vi "根据拍PCB孔点计算所有放料点.vi"(8 "放料点相对拍照点高度差(数组)":dbl[](array[numeric]), 9 "自动锁螺丝: 点位补偿值-单片PCB":T1[](array[typedef]), 11 "自动锁螺丝: PCB孔拍照点坐标-单片PCB":T2[](array[typedef])) -> (1 "放料点XYZ 数组":T1[](array[typedef]), 3 "放料点XYZR 数组":T3[](array[typedef]))   [LabVIEW 2014]
uses:
  Controls/XYZRPos.ctl
  Controls/XYZPos.ctl
  Global.vi
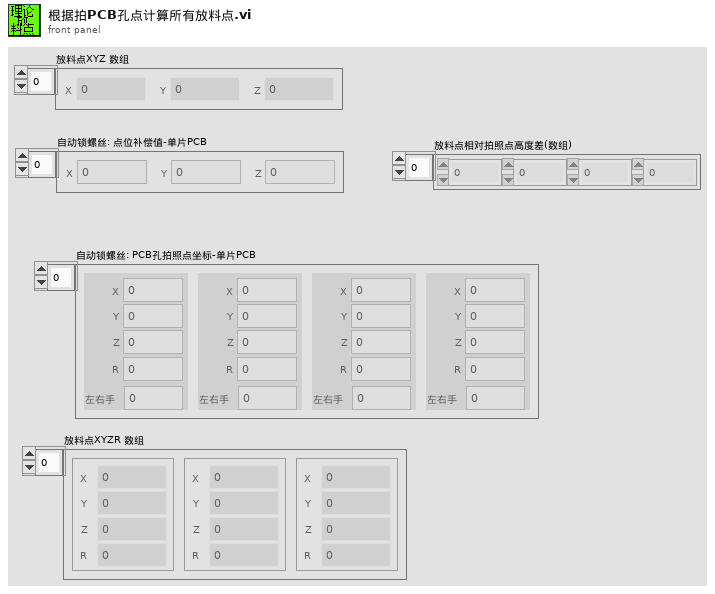
[diagram p1: front panel]
types:
  T1 = typedef "XYZPos.ctl" = cluster{"X":dbl, "Y":dbl, "Z":dbl}
  T2 = typedef "XYZRPos+左右手.ctl" = cluster{"坐标":T3, "左右手":dbl}
  T3 = typedef "XYZRPos.ctl" = cluster{"X":dbl, "Y":dbl, "Z":dbl, "R":dbl}
  T4 = typedef "XYPos.ctl" = cluster{"X":dbl, "Y":dbl}
  T5 = cluster{"[0]":dbl, "[1]":dbl, "[2]":dbl, "[3]":dbl}
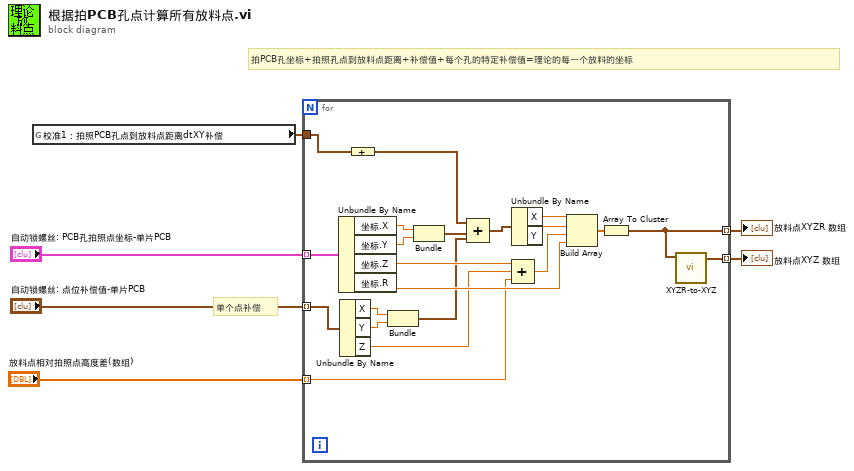
[diagram p0: block diagram]
diagram:
  # "拍PCB孔坐标+拍照孔点到放料点距离+补偿值+每个孔的特定补偿值=理论的每一个放料的坐标"
  # "单个点补偿"
  n1 = global read "Global.vi" "校准1：拍照PCB孔点到放料点距离dtXY补偿"() -> (w2:T4)
  n2 = for {
    tunnel: [w15] -> w6 mode=indexing
    tunnel: "自动锁螺丝: PCB孔拍照点坐标-单片PCB" -> [w21] mode=indexing
    tunnel: [w19] -> w5 mode=indexing
    tunnel: "自动锁螺丝: 点位补偿值-单片PCB" -> [w14] mode=indexing
    tunnel: w2 -> [w13]
    tunnel: "放料点相对拍照点高度差(数组)" -> [w7] mode=indexing
    n3 = Unbundle By Name(w21) -> ("坐标.X"=w27:dbl, "坐标.Y"=w26:dbl, "坐标.Z"=w17:dbl, "坐标.R"=w18:dbl)
    n4 = Unbundle By Name(w14) -> ("X"=w10:dbl, "Y"=w9:dbl, "Z"=w11:dbl)
    n5 = Compound Arithmetic op=unknown(w13) -> (w12:T4)
    n6 = Bundle("X"=w10, "Y"=w9) -> (w8:cluster{"X":dbl, "Y":dbl})  [unwired: 1 in]
    n7 = Bundle("X"=w27, "Y"=w26) -> (w25:cluster{"X":dbl, "Y":dbl})  [unwired: 1 in]
    n8 = Compound Arithmetic op=ADD(w12, w25, w8) -> (w20:T4)
    n9 = Unbundle By Name(w20) -> ("X"=w24:dbl, "Y"=w23:dbl)
    n10 = Compound Arithmetic op=ADD(w17, w11, w7) -> (w16:dbl)
    n11 = Build Array(w24, w23, w16, w18) -> (w22:dbl[])
    n12 = Array To Cluster(array=w22) -> (cluster=w15:T5)
    n13 = call "XYZR-to-XYZ.vi"("上相机拍照PCB孔时坐标P11"=w15) -> ("P-XYZ"=w19:T1)  [unwired: 10 in]
  }
  "放料点XYZR 数组" <- w6
  "放料点XYZ 数组" <- w5
